vi "Append Value to HHP.vi"(9 "Value":string, 10 "Key":string, 11 "HHP String In":string) -> (3 "HHP String Out":string)   [LabVIEW 2020, in "CHM Generator.lvclass"]
uses:
  CHM Generator.lvclass
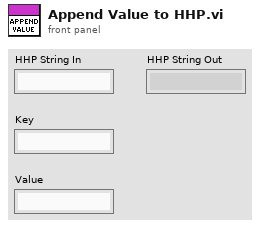
[diagram p1: front panel]
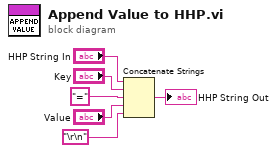
[diagram p0: block diagram]
diagram:
  n1 = Concatenate Strings("HHP String In", "Key", "=" ("string"), "Value", "\r\n") -> (→"HHP String Out":string)
